vi "告警信息文本转换为协议i12031值.vi"(11 "字符串":string) -> (3 "十进制整型字符串":string)   [LabVIEW 2016, in "数据传输系统-03.lvlib"]
panel:
  out "匹配子字符串":string
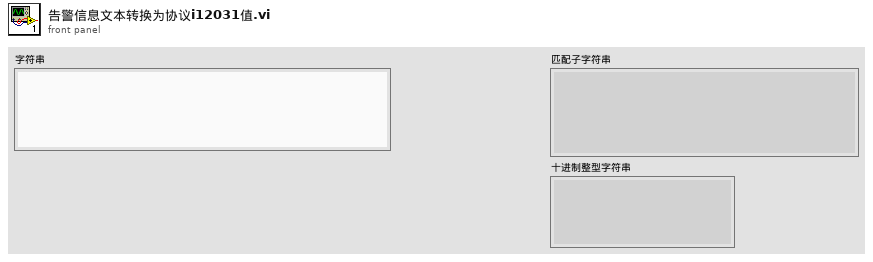
[diagram p1: front panel]
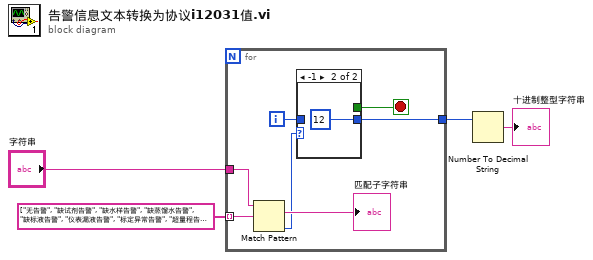
[diagram p0: block diagram]
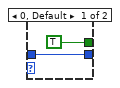
[diagram p2: hidden frame]
diagram:
  n1 = for {
    tunnel: [w7] -> w2
    tunnel: string[] ["无告警", "缺试剂告警", "缺水样告警", "缺蒸馏水告警", "缺标液告警", "仪表漏液告警", "标定异常告警", "超量程告警", "加热异常", "低试剂预警", "超上限告警", "超下限告警", "仪表内部其他异常", "滴定异常告警", "电极异常告警", "量程切换告警", "参数设置告警", "PH电极电位异常", "电导率电极异常", "浊度光度异常", "溶解氧电极异常", "溶解氧光强异常"] -> [w6] mode=indexing
    tunnel: "字符串" -> [w5]
    i -> [w8]
    stop <- w9 stop-if-true
    n2 = Match Pattern(string=w5, regular expression=w6) -> (match substring=→"匹配子字符串":string, offset past match=w10:i32)  [unwired: 1 in, 2 out]
    n3 = case shown="-1" w10 {
      tunnel: [TRUE _] -> w9
      tunnel: w8 -> [w12 _]
      tunnel: [w12 12] -> w7
      frame 0, Default {
      }
      frame -1 {
      }
    }
  }
  n4 = Number To Decimal String(number=w2) -> (decimal integer string=→"十进制整型字符串":string)  [unwired: 1 in]
